vi "subGetDestinationDir.vi"(9 "Project path":path, 11 "Refnum in":refnum<k20>) -> (1 "Name":string, 3 "Path":path)   [LabVIEW 2020, in "SolutionBuilder.lvlib"]
uses:
  SolutionBuilder.lvlib
  <vilib>/xml/NI_XML.lvlib
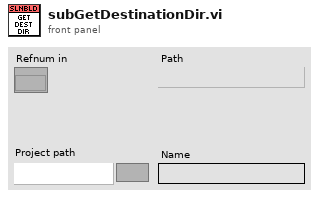
[diagram p1: front panel]
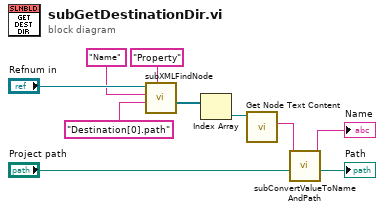
[diagram p0: block diagram]
diagram:
  n1 = call "subXMLFindNode.vi"("Node name"="Property", "Property value"="Destination[0].path", "Property name"="Name", "Refnum in"="Refnum in") -> ("Nodes"=w8:refnum<k20>[])  [unwired: 6 in, 1 out]
  n2 = Index Array(array=w8) -> (element=w9:refnum<k20>)  [unwired: 1 in]
  n3 = call <vilib>:"Get Node Text Content.vi"("node in"=w9) -> ("node text"=w3:string)  [unwired: 8 in, 2 out]
  n4 = call "subConvertValueToNameAndPath.vi"("Project path"="Project path", "Value"=w3) -> ("Path"=→"Path":path, "Name"=→"Name":string)  [unwired: 8 in]
